vi "外部调用接口全局变量.vi"() -> ()   [LabVIEW 2016]
panel:
  in  "数据库类型":T1
  in  "Password":string
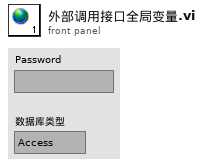
[diagram p1: front panel]
types:
  T1 = typedef "数据库类型.ctl" = enum16{"Access", "SQLite"}
diagram:
